vi "Update.vi"(8 "error in (no error)":errorcluster, 10 "Message in":refnum<class "UpdateMessage.lvclass">, 11 "wavefront sensor in":refnum<class "wavefront sensor.lvclass">) -> (0 "error out":errorcluster, 3 "wavefront sensor out":refnum<class "wavefront sensor.lvclass">)   [LabVIEW 2012, in "wavefront sensor.lvclass"]
doc: "The update method processes the command 'update'. \n\nThe command 'update' is used for receiving new values to be set to the private data of the class. This could be seen as a public set method for setting new parameters to the private class data."
uses:
  wavefront sensor.lvclass
  <vilib>/Distrio/Murmex/UpdateMessage/UpdateMessage.lvclass
  <vilib>/Distrio/Murmex/Murmex/Murmex.lvclass
panel:
  # "This method is called when the UPDATE\ntrigger is sent. \n\nOverride this method when your component needs to\nrespond to this trigger. \n\nCall parent for proper implementation"
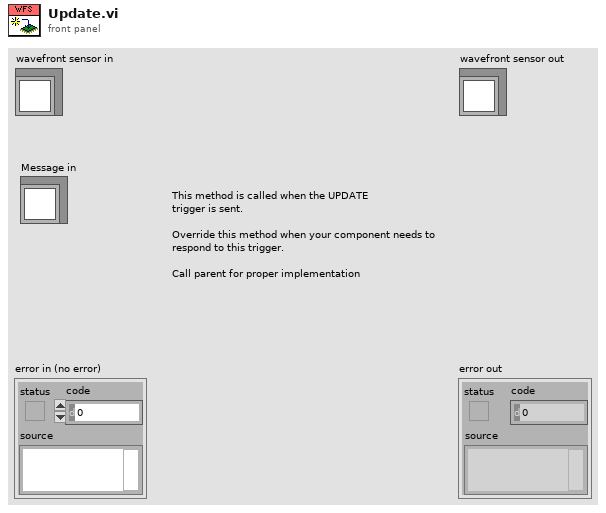
[diagram p1: front panel]
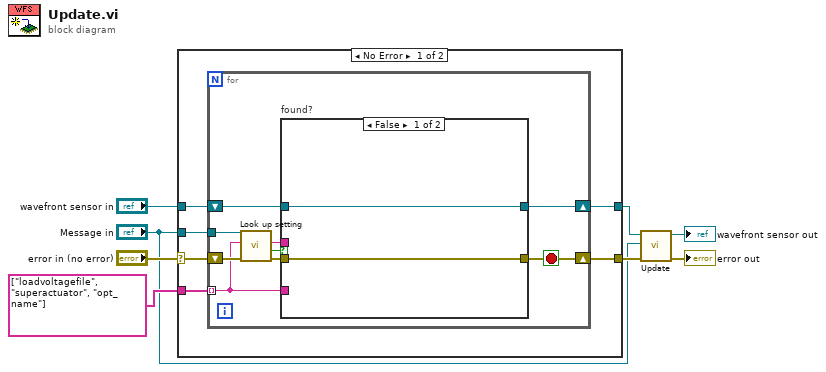
[diagram p0: block diagram]
diagram:
  n1 = case shown="No Error" "error in (no error)" {
    selector: "error in (no error)" -> [w14 w37]
    tunnel: "Message in" -> [w13 _]
    tunnel: "wavefront sensor in" -> [w12 w36]
    tunnel: string[] ["loadvoltagefile", "superactuator", "opt_name"] ("key chains") -> [w11 _]
    tunnel: [w10 w37] -> w3
    tunnel: [w9 w36] -> w2
    frame No Error {
      n2 = for {
        shift-right: [w15] -> w10
        shift-left: w14 -> [w23]
        tunnel: w13 -> [w22]
        shift-right: [w17] -> w9
        shift-left: w12 -> [w19]
        tunnel: w11 -> [w16] mode=indexing
        stop <- w15 stop-if-true
        n3 = call <vilib>:"Look up setting.vi"("error in (no error)"=w23, "tag name"=w16, "UpdateMessage in"=w22) -> ("error out"=w21:errorcluster, "found?"=w20:bool, "value"=w18:string)  [unwired: 5 in, 1 out]
        n4 = case "found?" shown="False" w20 {
          tunnel: w21 -> [w24 w30]
          tunnel: w19 -> [w25 w28]
          tunnel: w18 -> [_ w31]
          tunnel: [w24 w29] -> w15
          tunnel: [w25 w27] -> w17
          tunnel: w16 -> [_ w26]
          frame False {
          }
          frame True {
            n5 = case "setting" shown="\"False\", Default" w26 {
              tunnel: w31 -> [_ _]
              tunnel: w30 -> [w32 w35]
              tunnel: [w32 w35] -> w29
              tunnel: w28 -> [w33 w34]
              tunnel: [w33 w34] -> w27
              frame "False", Default {
              }
              frame "True" {
              }
            }
          }
        }
      }
    }
    frame Error {
    }
  }
  n6 = call-parent "Update.vi"("error in (no error)"=w3, "Message in"="Message in", "Murmex in"=w2) -> ("error out"=→"error out":errorcluster, "Murmex out"=→"wavefront sensor out":refnum<class "wavefront sensor.lvclass">)  [unwired: 7 in]
